vi "Speed.vi"(0 "Comport":refnum<visa-resource-name>, 1 "Speed":i32, 2 "SPD":i32=43, 3 "INCR":i32=40, 4 "STPS":i32=10) -> ()   [LabVIEW 2016]
uses:
  <vilib>/Instr/_visa.llb/VISA Configure Serial Port (Instr).vi
panel:
  out "Set Success":bool
  # "Steps/Sec"
  # "Steps/Sec"
  # "Maximum speed 4000 Microns/Sec"
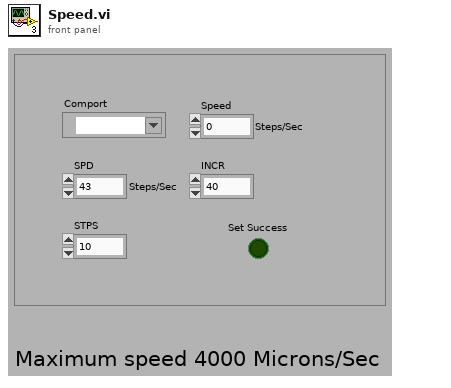
[diagram p1: front panel]
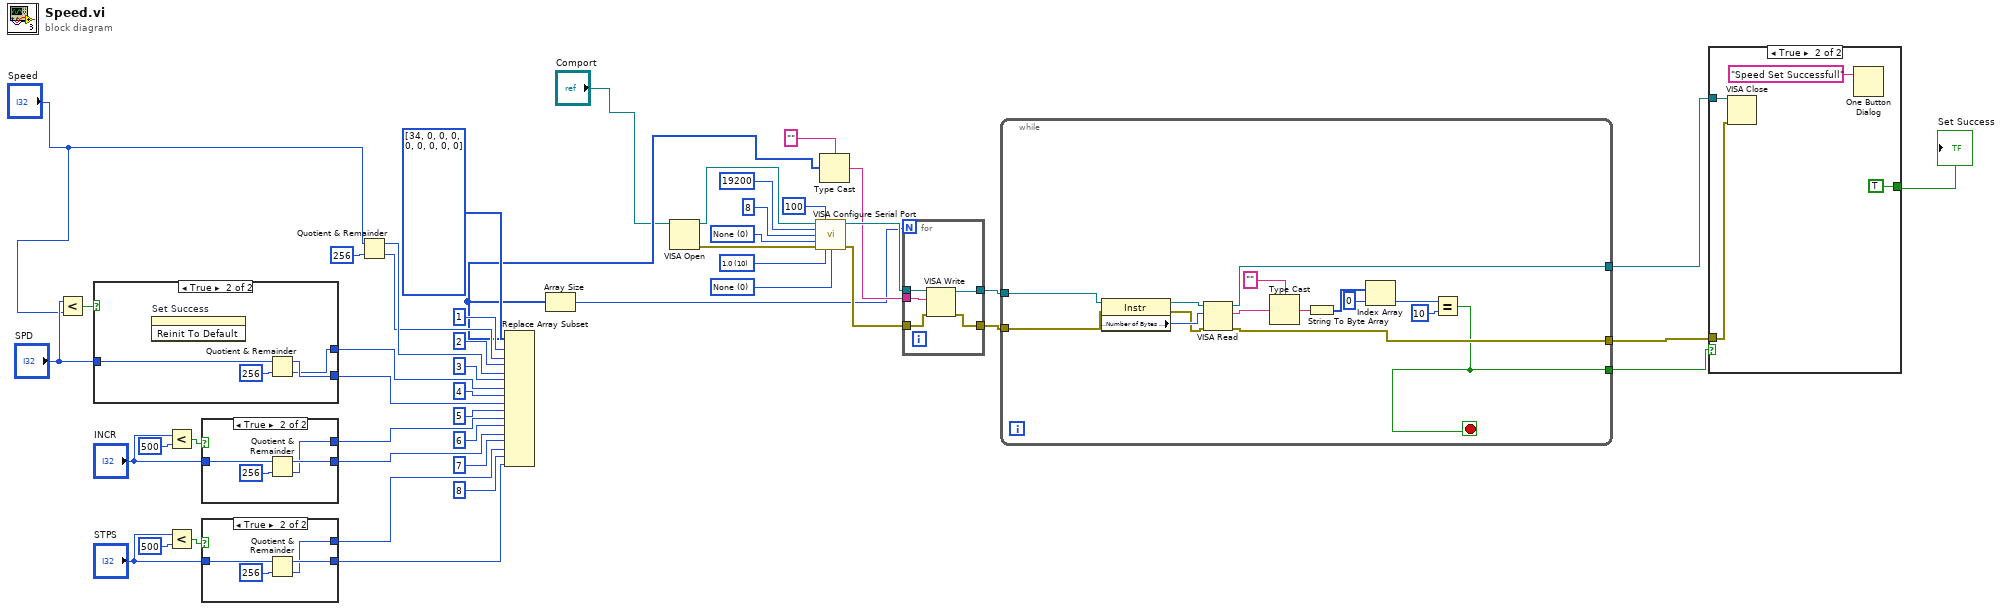
[diagram p0: block diagram]
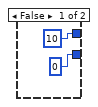
[diagram p2: hidden frame]
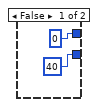
[diagram p3: hidden frame]
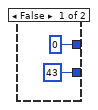
[diagram p4: hidden frame]
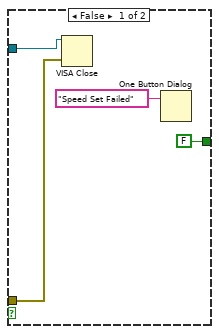
[diagram p5: hidden frame]
diagram:
  w10 = u16 0 items=["None"=0, "XON/XOFF"=1, "RTS/CTS"=2, "DTR/DSR"=4] ("flow control")
  w11 = u16 10 items=["1.0"=10, "1.5"=15, "2.0"=20] ("stop bits")
  w12 = u16 0 items=["None", "Odd", "Even", "Mark", "Space"] ("parity")
  n1 = Less?(x="SPD", y="Speed") -> (x < y?=w32:bool)
  n2 = case shown="True" w32 {
    tunnel: "SPD" -> [_ w54]
    tunnel: [43 w52] -> w42
    tunnel: [u16 0 w51] -> w41
    frame False {
    }
    frame True {
      n3 = invoke on="Set Success" class="Bool (strict)" method="Reinit To Default"() -> ()  [unwired: 3 in, 3 out]
      n4 = Quotient & Remainder(x=w54, y=u16 256) -> (x-y*floor(x/y)=w52:i32, floor(x/y)=w51:i32)
    }
  }
  n5 = Less?(x="INCR", y=u16 500) -> (x < y?=w35:bool)
  n6 = Less?(x="STPS", y=u16 500) -> (x < y?=w36:bool)
  n7 = case shown="True" w35 {
    tunnel: "INCR" -> [_ w60]
    tunnel: [40 w59] -> w46
    tunnel: [u16 0 w57] -> w43
    frame False {
    }
    frame True {
      n8 = Quotient & Remainder(x=w60, y=u16 256) -> (x-y*floor(x/y)=w59:i32, floor(x/y)=w57:i32)
    }
  }
  n9 = case shown="True" w36 {
    tunnel: "STPS" -> [_ w64]
    tunnel: [u16 0 w66] -> w47
    tunnel: [10 w63] -> w48
    frame False {
    }
    frame True {
      n10 = Quotient & Remainder(x=w64, y=u16 256) -> (x-y*floor(x/y)=w66:i32, floor(x/y)=w63:i32)
    }
  }
  n11 = Quotient & Remainder(x="Speed", y=u32 256) -> (x-y*floor(x/y)=w40:u32, floor(x/y)=w22:u32)
  n12 = Replace Array Subset(array=u8[] [34, 0, 0, 0, 0, 0, 0, 0, 0], new element #1=w22, index #1=1 ("index"), new element #2=w40, index #2=2 ("index"), new element #3=w41, index #3=3 ("index"), new element #4=w42, index #4=4 ("index"), new element #5=w43, index #5=5 ("index"), new element #6=w46, index #6=6 ("index"), new element #7=w48, index #7=7 ("index"), new element #8=w47, index #8=8 ("index")) -> (w19:u8[])
  n13 = Array Size(array=w19) -> (size(s)=w2:i32)
  n14 = VISA Open(VISA resource name="Comport") -> (VISA resource name=w5:refnum<visa-resource-name>, error out=w4:errorcluster)  [unwired: 4 in]
  n15 = call-poly "VISA Configure Serial Port"("VISA resource name"=w5, "timeout (10sec)"=u32 100, "baud rate (9600)"=u32 19200 ("baud rate"), "data bits (8)"=u16 8 ("data bits"), "parity (0:none)"=w12, "error in (no error)"=w4, "stop bits (10: 1 bit)"=w11, "flow control (0:none)"=w10) -> ("VISA resource name out"=w13:refnum<visa-resource-name>, "error out"=w14:errorcluster)  [unwired: 1 in, 5 out]
  n16 = Type Cast(type="", x=w19) -> (*(type *) &x=w8:string)
  n17 = for {
    N: w2 -> [_]
    tunnel: w8 -> [w67]
    tunnel: w13 -> [w68]
    tunnel: [w70] -> w16
    tunnel: w14 -> [w69]
    tunnel: [w71] -> w17
    n18 = VISA Write(VISA resource name=w68, write buffer=w67, error in (no error)=w69) -> (VISA resource name out=w70:refnum<visa-resource-name>, error out=w71:errorcluster)  [unwired: 1 out]
  }
  n19 = while {
    tunnel: [w86] -> w21
    tunnel: w16 -> [w77]
    tunnel: w17 -> [w76]
    tunnel: [w85] -> w20
    tunnel: [w72] -> w18
    stop <- w72 stop-if-true
    n20 = property class="Instr"(reference=w77, error in=w76) -> (reference out=w75:refnum<visa-resource-name>, error out=w73:errorcluster, "Serial Settings:Number of Bytes at Serial Port"=w74:u32)
    n21 = VISA Read(VISA resource name=w75, byte count=w74, error in (no error)=w73) -> (VISA resource name out=w86:refnum<visa-resource-name>, read buffer=w84:string, error out=w85:errorcluster)  [unwired: 1 out]
    n22 = Type Cast(type="", x=w84) -> (*(type *) &x=w82:string)
    n23 = String To Byte Array(string=w82) -> (unsigned byte array=w81:u8[])
    n24 = Index Array(array=w81, index=0) -> (element=w79:u8)
    n25 = Equal?(x=w79, y=u8 10) -> (x = y?=w72:bool)
  }
  n26 = case shown="True" w18 {
    tunnel: [FALSE TRUE] -> w23
    tunnel: w21 -> [w88 w92]
    tunnel: w20 -> [w87 w91]
    frame False {
      n27 = VISA Close(VISA resource name=w88, error in (no error)=w87) -> ()  [unwired: 1 out]
      n28 = One Button Dialog(message="Speed Set Failed") -> ()  [unwired: 1 in, 1 out]
    }
    frame True {
      n29 = VISA Close(VISA resource name=w92, error in (no error)=w91) -> ()  [unwired: 1 out]
      n30 = One Button Dialog(message="Speed Set Successfull") -> ()  [unwired: 1 in, 1 out]
    }
  }
  "Set Success" <- w23
